vi "DAQmx Task and Channel  2 Channel.vi"(9 "Channel Path List In":string[](array[string]), 10 "Channel In":string, 11 "DAQmx Task Name":refnum<k21>) -> (1 "Channel Name Index":i32, 3 "Channel Out":string, 4 "Exists":bool)   [LabVIEW 2013]
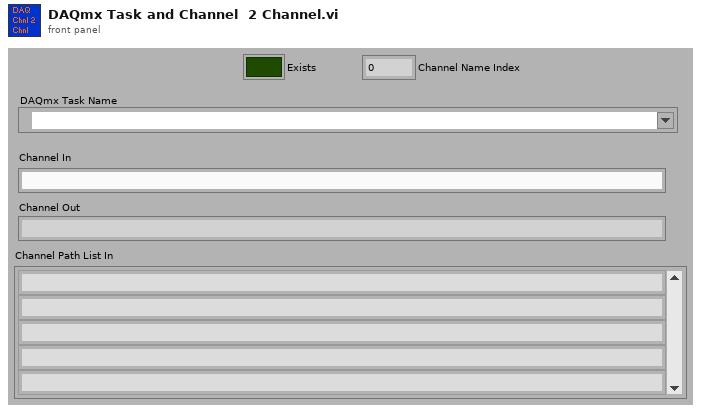
[diagram p1: front panel]
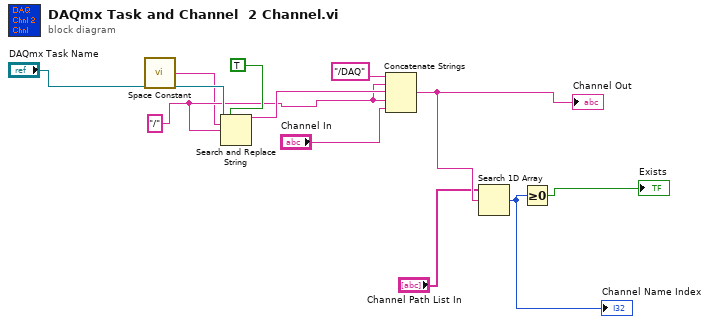
[diagram p0: block diagram]
diagram:
  w8 = "/"
  n1 = call <vilib>:"Space Constant.vi"() -> ("String"=w7:string)
  n2 = Search and Replace String(replace all?=TRUE ("replace all? (F)"), input string="DAQmx Task Name", search string=w7, replace string=w8) -> (result string=w9:string)  [unwired: 1 in, 6 out]
  n3 = Concatenate Strings("/DAQ" ("string"), w8, w9, w8, "Channel In") -> (w4:string)
  "Channel Out" <- w4
  n4 = Search 1D Array(1D array="Channel Path List In", element=w4) -> (index of element=w2:i32)  [unwired: 1 in]
  "Channel Name Index" <- w2
  n5 = Greater Or Equal To 0?(x=w2) -> (x >= 0?=→"Exists":bool)
